vi "图像处理1.vi"(0 "Image In":T1, 7 "error in":errorcluster, 8 "系数":sgl, 10 "偏置":sgl) -> (18 "时间":sgl, 20 "Image Out":T1)   [LabVIEW 2014]
uses:
  <vilib>/vision/Image Controls.llb/IMAQ Image.ctl
  <vilib>/vision/NI_Vision_Development_Module.lvlib
panel:
  out "Image Out 2":T1
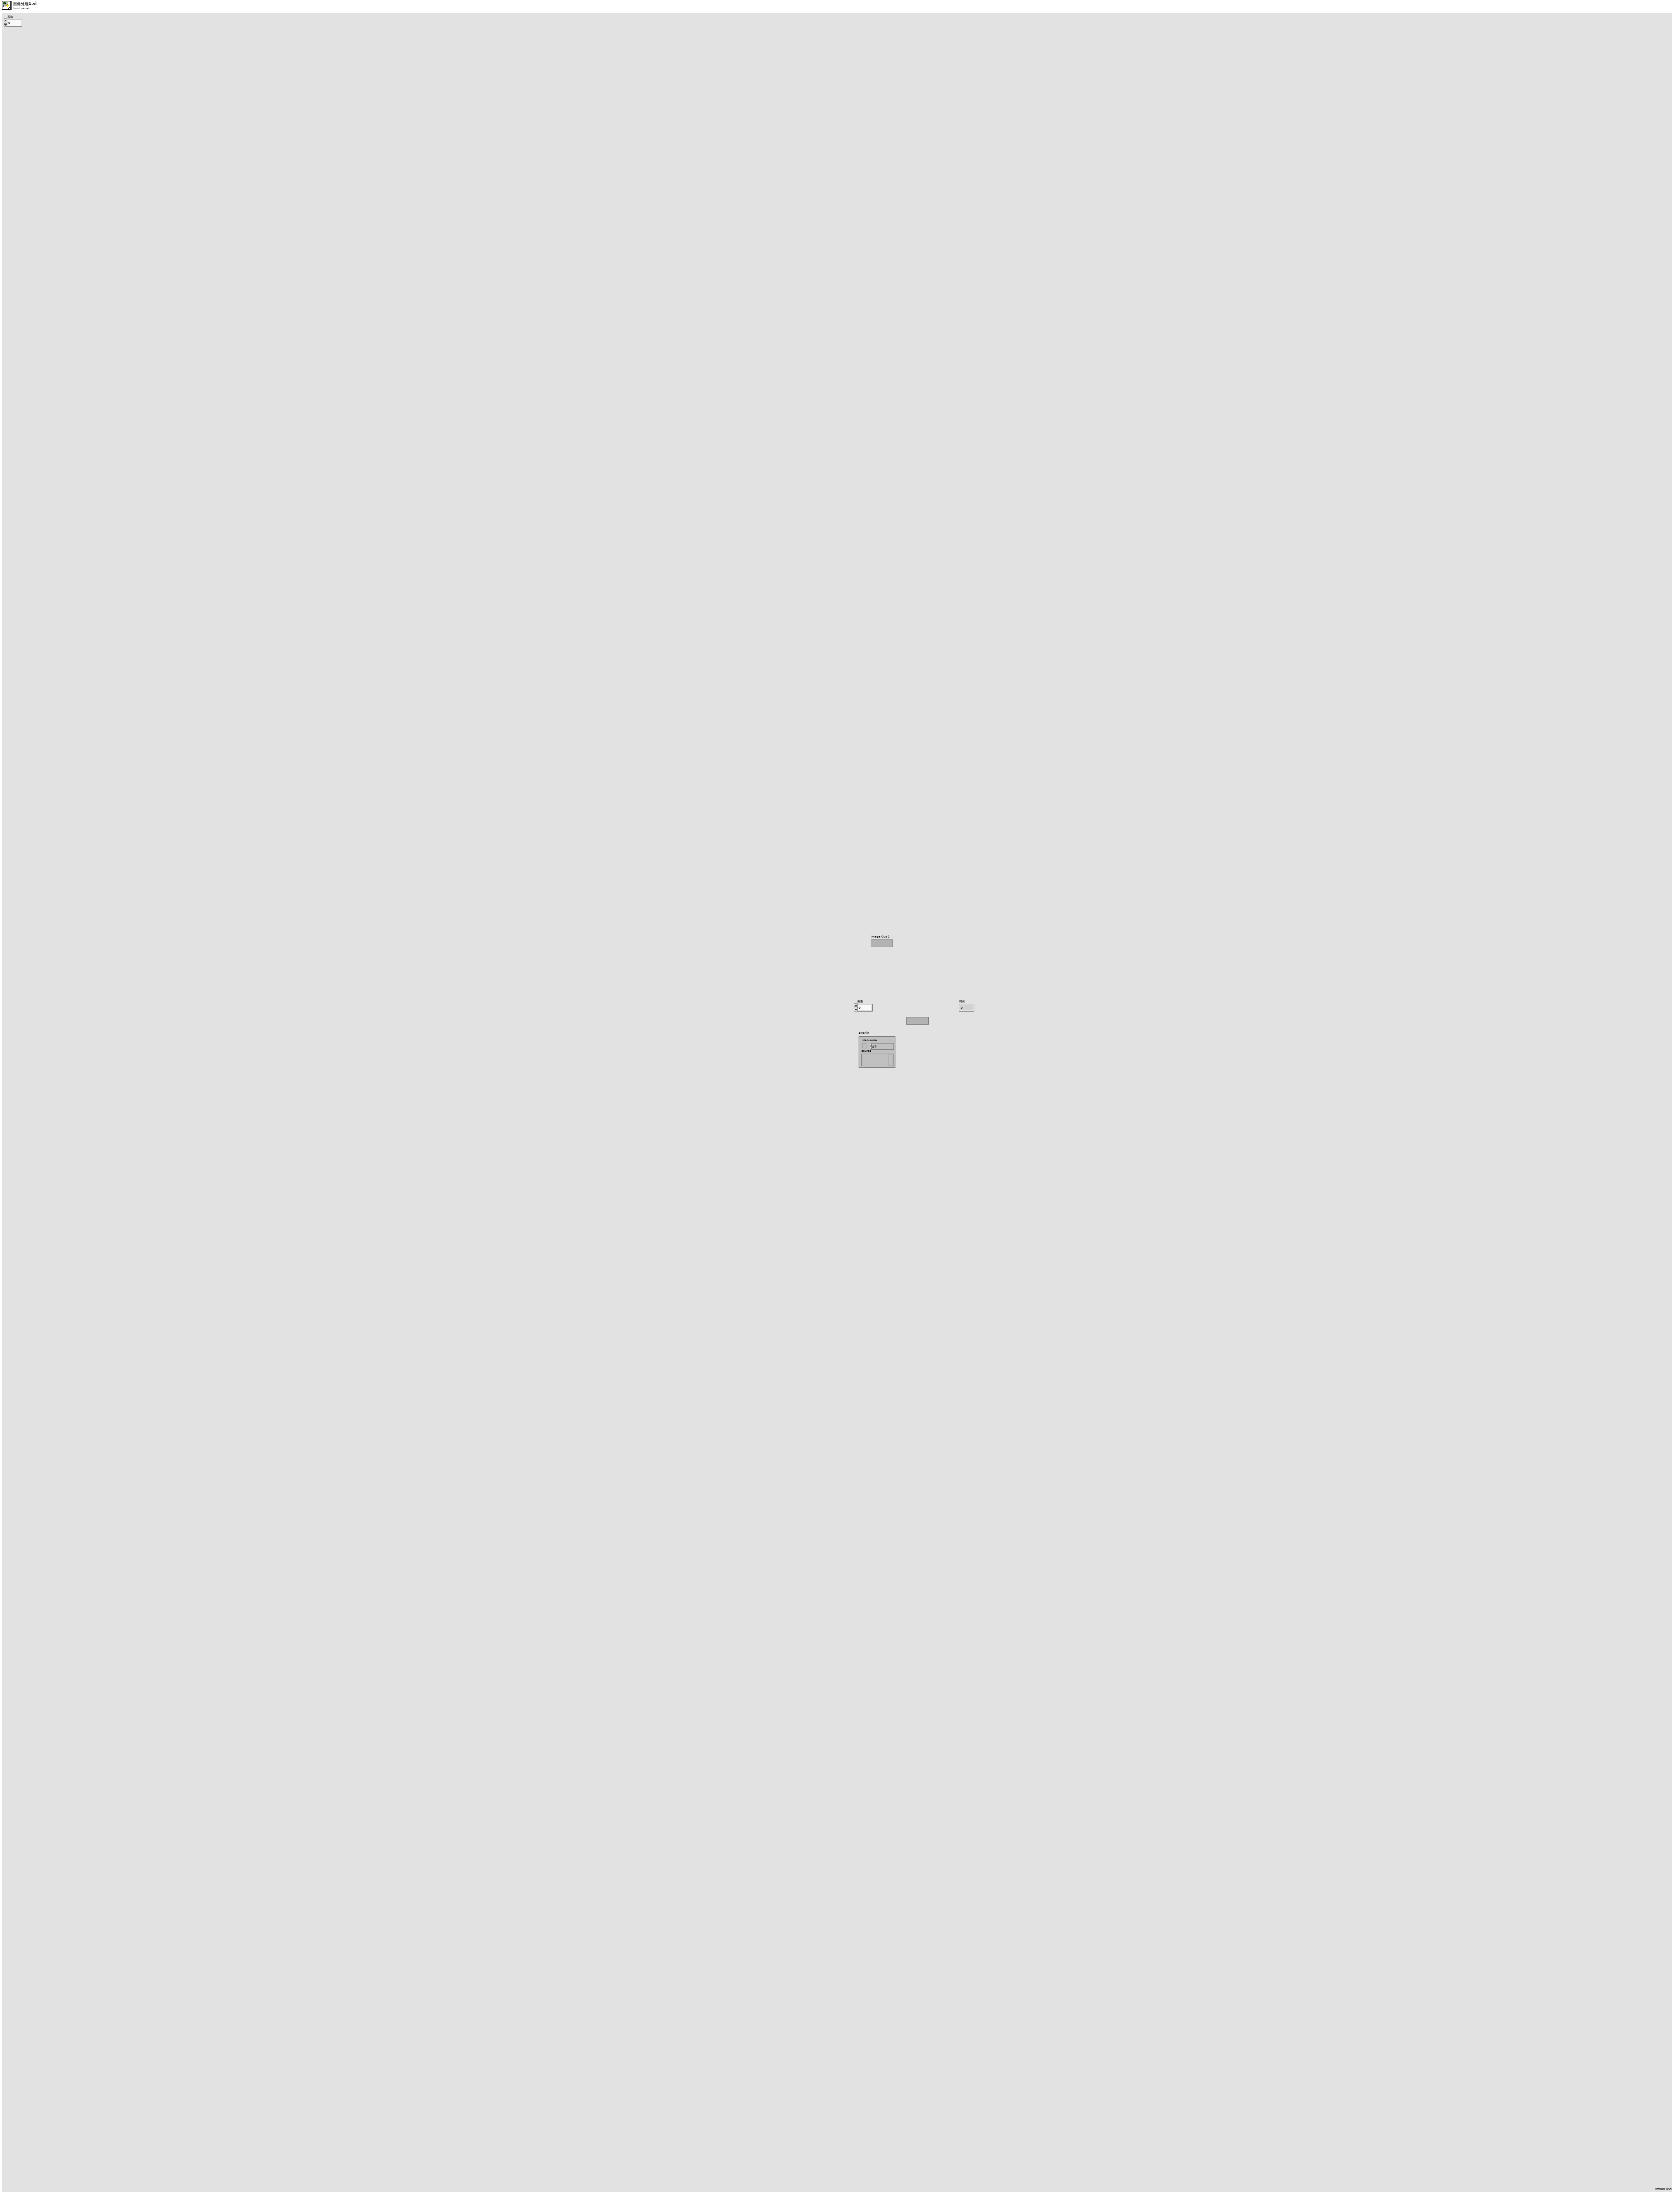
[diagram p1: front panel]
types:
  T1 = typedef "IMAQ Image.ctl" = refnum<image>
  T2 = cluster{"Measurement Parameter":i32, "Range Lower Value":dbl, "Range Upper Value":dbl, "Range":bool, "Measurement Type":bool}[]
  T3 = typedef "IMAQ Rectangle" = cluster{"Left":i32, "Top":i32, "Right":i32, "Bottom":i32, "Rotation":dbl}
  T4 = cluster{"Sigma":sgl, "HThresh":sgl, "LThres":sgl, "WindowSize":i32}
  T5 = cluster{"Number of Matches Requested":i32, "Minimum Match Score":sgl, "Angle Ranges":cluster{"Start Angle":sgl, "End Angle":sgl}[]}
  T6 = cluster{"Global Rectangle":i32[], "Contours":cluster{"ID":enum32{"External", "Internal"}, "Type":u32, "Coordinates":i32[]}[]}
  T7 = cluster{"Position":cluster{"x":sgl, "y":sgl}, "Angle":sgl, "Scale":sgl, "Score":sgl, "Bounding Box":cluster{"x":sgl, "y":sgl}[]}[]
  T8 = typedef "ROI Descriptor" = cluster{"Global Rectangle":i32[], "Contours":cluster{"ID":enum32{"External", "Internal"}, "Type":u32, "Coordinates":i32[]}[]}
  T9 = cluster{"Position":cluster{"x":sgl, "y":sgl}, "Angle":sgl, "Scale":sgl, "Score":sgl, "Bounding Box":cluster{"x":sgl, "y":sgl}[]}
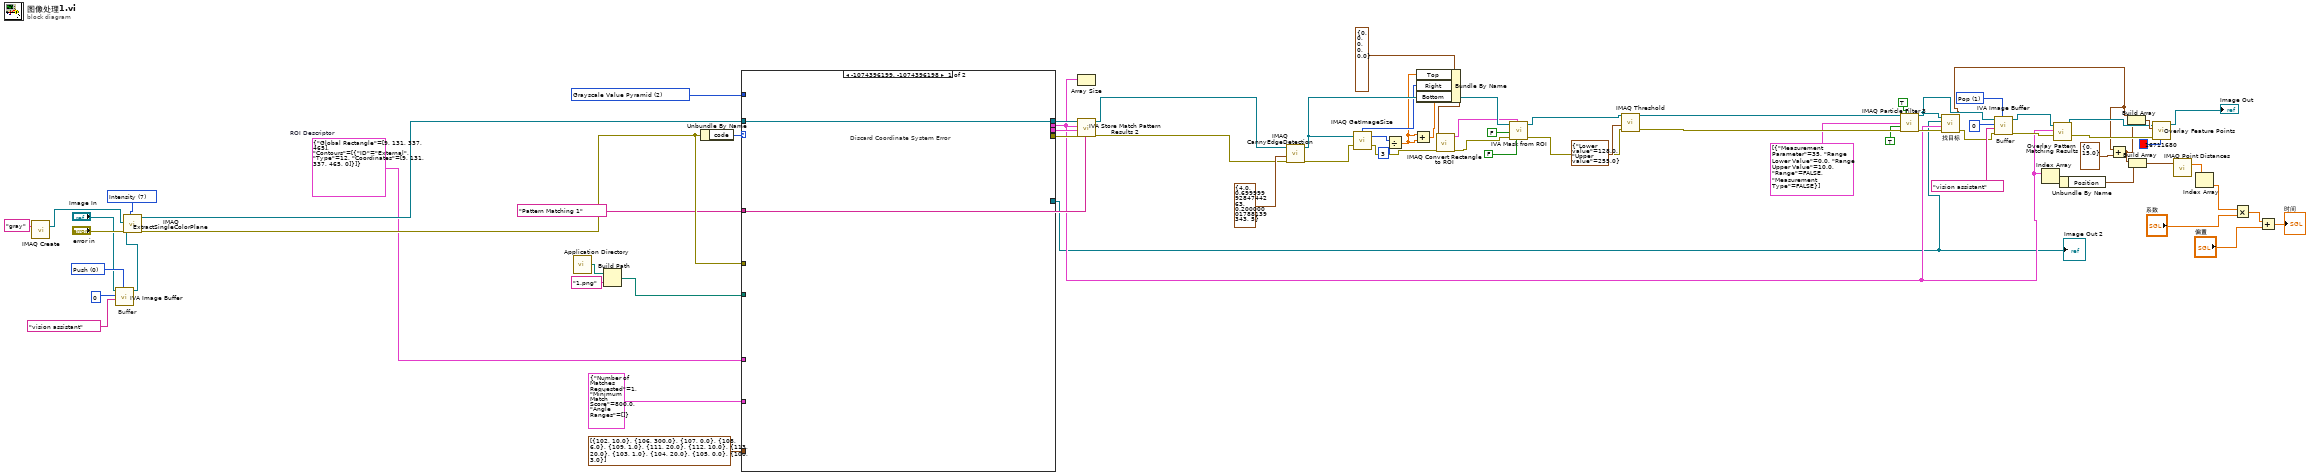
[diagram p0: block diagram]
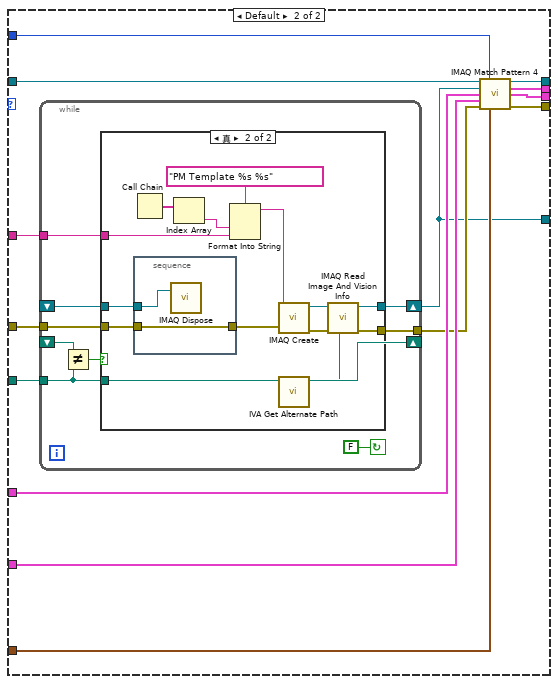
[diagram p2: hidden frame]
diagram:
  w26 = u16 1 items=["Push", "Pop", "Reset"] ("Function")
  w59 = u16 0 items=["Push", "Pop", "Reset"] ("Function")
  w67 = 2 items=["All", "Low Discrepancy Sampling", "Grayscale Value Pyramid", "Gradients Pyramid"] ("Algorithm")
  w63 = "Pattern Matching 1" ("Step Name")
  w66 = T6 {"Global Rectangle"=[9, 131, 337, 465], "Contours"=[{"ID"=enum."External", "Type"=12, "Coordinates"=[9, 131, 337, 465, 0]}]}  # ROI Descriptor
  w74 = 7 items=["Red", "Green", "Blue", "Hue", "Saturation", "Luminance", "Value", "Intensity"] ("Color Plane")
  # "Buffer"
  # "Buffer"
  n1 = call "IMAQ Create"("Image Name"="gray") -> ("New Image"=w60:T1)  [unwired: 4 in, 1 out]
  n2 = call <vilib>:"IVA Image Buffer.vi"("Function"=w59, "Prefix"="vision assistant", "Buffer #"=0, "Image In"="Image In") -> ("Image Out"=w55:T1)  [unwired: 1 in, 6 out]
  n3 = call "IMAQ ExtractSingleColorPlane"("Color Plane"=w74, "error in (no error)"="error in", "Image Dst"=w60, "Image Src"=w55) -> ("error out"=w72:errorcluster, "Image Dst Out"=w71:T1)  [unwired: 6 out]
  n4 = call <vilib>:"Application Directory.vi"() -> ("Application Directory"=w54:path)
  n5 = Build Path(base path=w54, name or relative path="1.png" ("名称或相对路径")) -> (appended path=w52:path)
  n6 = Unbundle By Name(w72) -> ("code"=w68:i32)
  n7 = case "条件结构" shown="-1074396199, -1074396198" w68 {
    tunnel: w52 -> [_ w89]
    tunnel: w72 -> [_ w88]
    tunnel: w71 -> [w75 w84]
    tunnel: [_ w85] -> w70
    tunnel: [_ w86] -> w7
    tunnel: [w75 w83] -> w69
    tunnel: w63 -> [_ w87]
    tunnel: w67 -> [_ w82]
    tunnel: w66 -> [_ w81]
    tunnel: T5 {"Number of Matches Requested"=1, "Minimum Match Score"=800.0, "Angle Ranges"=[]} ("Parameters") -> [_ w80]
    tunnel: cluster{"Item":u16, "Value":dbl}[] [{"Item"=102, "Value"=10.0}, {"Item"=106, "Value"=300.0}, {"Item"=107, "Value"=0.0}, {"Item"=108, "Value"=6.0}, {"Item"=109, "Value"=1.0}, {"Item"=111, "Value"=20.0}, {"Item"=112, "Value"=10.0}, {"Item"=113, "Value"=20.0}, {"Item"=103, "Value"=1.0}, {"Item"=104, "Value"=20.0}, {"Item"=105, "Value"=0.0}, {"Item"=100, "Value"=3.0}] ("Advanced Options") -> [_ w78]
    tunnel: [_ w77] -> w62
    tunnel: [_ w76] -> w6
    frame -1074396199, -1074396198 {
      # "Discard Coordinate System Error"
    }
    frame Default {
      n8 = while {
        shift-right: [w98] -> w76
        shift-left: _ -> [w97]
        tunnel: [w95] -> w79
        tunnel: w88 -> [w94]
        tunnel: w89 -> [w91]
        tunnel: w87 -> [w93]
        shift-right: [w91] -> _
        shift-left: _ -> [w92]
        stop <- FALSE continue-if-true
        n9 = Not Equal?(x=w92, y=w91) -> (x != y?=w90:bool)
        n10 = case "条件结构" shown="真" w90 {
          tunnel: [w100 w112] -> w98
          tunnel: w97 -> [w100 w103]
          tunnel: [w99 w109] -> w95
          tunnel: w94 -> [w99 w102]
          tunnel: w91 -> [_ w105]
          tunnel: w93 -> [_ w106]
          frame False {
          }
          frame True {
            n11 = stacked-sequence "层叠式顺序结构" {
              tunnel: w103 -> [w116]
              tunnel: w102 -> [w115]
              tunnel: [w115] -> w101
              frame #0 {
                n12 = call "IMAQ Dispose"("Image"=w116) -> ()  [unwired: 2 in, 4 out]
              }
            }
            n13 = Call Chain() -> (call chain=w108:string[])
            n14 = Index Array(array=w108) -> (element=w107:string)  [unwired: 1 in]
            n15 = Format Into String(format string="PM Template %s %s" ("Image Name"), w107, w106) -> (resulting string=w114:string)  [unwired: 2 in, 1 out]
            n16 = call "IMAQ Create"("Image Name"=w114, "error in (no error)"=w101) -> ("New Image"=w111:T1, "error out"=w110:errorcluster)  [unwired: 2 in, 1 out]
            n17 = call <vilib>:"IVA Get Alternate Path.vi"("Path In"=w105) -> ("Path Out"=w104:path)  [unwired: 10 out]
            n18 = call "IMAQ Read Image And Vision Info"("File Path"=w104, "error in (no error)"=w110, "Image"=w111) -> ("error out"=w109:errorcluster, "Image Out"=w112:T1)  [unwired: 1 in, 6 out]
          }
        }
      }
      n19 = call "IMAQ Match Pattern 4"("Image"=w84, "Algorithm"=w82, "Template Image"=w76, "ROI Descriptor"=w81, "Parameters"=w80, "error in (no error)"=w79, "Advanced Options"=w78) -> ("Image (duplicate)"=w83:T1, "Matches (pixel)"=w86:T7, "Matches (real-world)"=w77:T7, "error out"=w85:errorcluster)  [unwired: 4 in, 1 out]
    }
  }
  "Image Out 2" <- w6
  n20 = Array Size(array=w7) -> ()  [unwired: 1 out]
  n21 = call <vilib>:"IVA Store Match Pattern Results 2.vi"("Step Name"=w63, "error in (no error)"=w70, "Matches (real-world)"=w62, "Matches (pixel)"=w7, "Image in"=w69) -> ("error out"=w50:errorcluster, "Image dup"=w49:T1)  [unwired: 1 in, 4 out]
  n22 = call "IMAQ CannyEdgeDetection"("Image Src"=w49, "Filter Parameters"=T4 {"Sigma"=4.0, "HThresh"=0.6999999, "LThres"=0.20000002, "WindowSize"=5}, "error in (no error)"=w50) -> ("Image Dst Out"=w46:T1, "error out"=w45:errorcluster)  [unwired: 1 in, 4 out]
  n23 = call "IMAQ GetImageSize"("Image"=w46, "error in (no error)"=w45) -> ("Y Resolution"=w42:i32, "X Resolution"=w39:i32, "error out"=w44:errorcluster)  [unwired: 2 in]
  n24 = Divide(x=w42, y=3) -> (x/y=w38:dbl)
  n25 = Add(x=w38, y=w38) -> (x+y=w37:dbl)
  n26 = Bundle By Name(cluster=T3 {"Left"=0, "Top"=0, "Right"=0, "Bottom"=0, "Rotation"=0.0} ("Rectangle"), "Top"=w38, "Right"=w39, "Bottom"=w37) -> (w36:T3)
  n27 = call "IMAQ Convert Rectangle to ROI"("error in (no error)"=w44, "Rectangle"=w36) -> ("error out"=w43:errorcluster, "ROI Descriptor"=w35:T8)  [unwired: 7 in]
  n28 = call <vilib>:"IVA Mask from ROI.vi"("Shrink"=FALSE, "ROI Descriptor"=w35, "error in (no error)"=w43, "Out / In"=FALSE, "Image Src"=w46) -> ("error out"=w27:errorcluster, "Image Out"=w28:T1)  [unwired: 1 in, 4 out]
  n29 = call "IMAQ Threshold"("error in (no error)"=w27, "Range"=cluster{"Lower value":sgl, "Upper value":sgl} {"Lower value"=128.0, "Upper value"=255.0}, "Image Src"=w28) -> ("error out"=w33:errorcluster, "Image Dst Out"=w30:T1)  [unwired: 3 in, 4 out]
  n30 = call "IMAQ Particle Filter 3"("Image Src"=w30, "Connectivity 4/8 (8)"=TRUE, "Selection Values"=T2 [{"Measurement Parameter"=35, "Range Lower Value"=0.0, "Range Upper Value"=10.0, "Range"=FALSE, "Measurement Type"=FALSE}], "Keep/Remove Particles (F)"=TRUE ("Keep/Remove Particles"), "error in (no error)"=w33) -> ("Image Dst Out"=w21:T1, "error out"=w23:errorcluster)  [unwired: 4 in, 5 out]
  n31 = call "找目标.vi"("error in (no error)"=w23, "Matches (pixel)"=w7, "temp"=w6, "Image"=w21) -> ("error out"=w22:errorcluster, "目标点"=w1:cluster{i32, dbl})  [unwired: 5 in, 1 out]
  n32 = call <vilib>:"IVA Image Buffer.vi"("Function"=w26, "error in (no error)"=w22, "Prefix"="vision assistant", "Buffer #"=0, "Image In"=w21) -> ("error out"=w8:errorcluster, "Image Out"=w20:T1)  [unwired: 5 out]
  n33 = Index Array(array=w7) -> (element=w16:T9)  [unwired: 1 in]
  n34 = call "Overlay Pattern Matching Results.vi"("Matches"=w7, "Image"=w20) -> ("Image Out"=w9:T1)  [unwired: 8 in, 1 out]
  n35 = Unbundle By Name(w16) -> ("Position"=w2:cluster{"x":sgl, "y":sgl})
  n36 = Add(x=w1, y=cluster{i32, dbl} {0, 15.0}) -> (x+y=w3:cluster{i32, dbl})
  n37 = Build Array(w1, w3) -> (w19:cluster{i32, dbl}[])
  n38 = Build Array(w3, w2) -> (w17:cluster{"x":sgl, "y":dbl}[])
  n39 = call "Overlay Feature Points.vi"("Color"=u32 16711680, "error in"=w8, "Feature Points"=w19, "Image"=w9) -> ("Image Out"=→"Image Out":T1)  [unwired: 6 in, 1 out]
  n40 = call "IMAQ Point Distances"("Points"=w17) -> ("Distances"=w14:sgl[])  [unwired: 4 in, 1 out]
  n41 = Index Array(array=w14) -> (element=w13:sgl)  [unwired: 1 in]
  n42 = Multiply(x=w13, y="系数") -> (x*y=w12:sgl)
  n43 = Add(x=w12, y="偏置") -> (x+y=→"时间":sgl)
